vi "Finish.vi"   [LabVIEW 2013]
doc: "This VI is called just before exiting. It is expected to close I/O refnum, save collected data, etc."
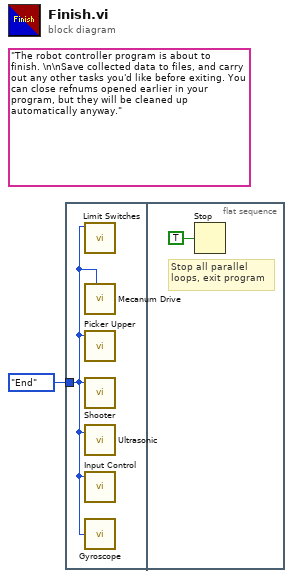
[diagram p0: block diagram]
diagram:
  (unwired) "The robot controller program is about to finish. \n\nSave collected data to files, and carry out any other tasks you'd like before exiting. You can close refnums opened earlier in your program, but they will be cleaned up automatically anyway."
  n1 = flat-sequence {
    tunnel: enum16{"Open", "Run", "End"}."End" ("State Control") -> [w2]
    frame #0 {
      n2 = call "Limit Switches.vi"("State Control"=w2) -> ()  [unwired: 7 in, 4 out]
      n3 = call "Mecanum Drive.vi"("State Control"=w2) -> ()  [unwired: 5 in]
      n4 = call "Picker Upper.vi"("State Control"=w2) -> ()  [unwired: 2 in]
      n5 = call "Shooter.vi"("State Control"=w2) -> ()  [unwired: 2 in]
      n6 = call "Ultrasonic.vi"("State Control"=w2) -> ()  [unwired: 2 in]
      n7 = call "Input Control.vi"("State"=w2) -> ()  [unwired: 2 in, 3 out]
      n8 = call "Gyroscope.vi"("State Control"=w2) -> ()  [unwired: 2 out]
    }
    frame #1 {
      # "Stop all parallel\nloops, exit program"
      n9 = Stop(stop? (T)=TRUE ("Quit")) -> ()
    }
  }
